vi "Load VI for Subpanel.vi"() -> (2 "VI Path":path, 3 "VI out":refnum<vi>)   [LabVIEW 2021, in "TSC Button Editor.lvclass"]
doc: "This VI loads in the subpanel VI at program start which contains a sample Boolean control.\n\n<b>Code Developed By:</b>\nTechnology Service Corporation\nwww.tsc.com/atcs\n\nDeveloper:\nDaniel Coons"
uses:
  TSC Button Editor.lvclass
  TSC Button Editor.lvclass/TSC Button Editor.ctl
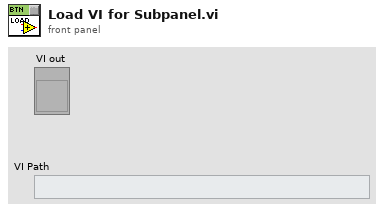
[diagram p1: front panel]
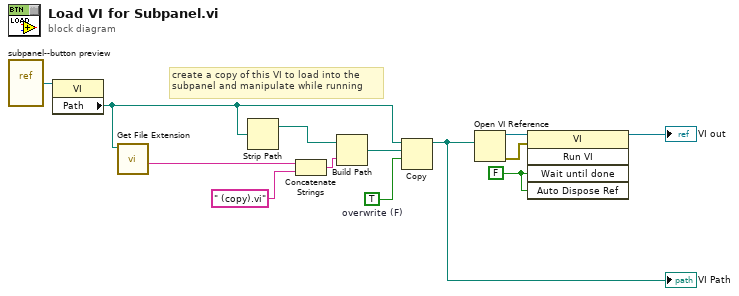
[diagram p0: block diagram]
diagram:
  w4 = TRUE  # overwrite (F)
  w2 = FALSE ("Activate?")
  # "create a copy of this VI to load into the \nsubpanel and manipulate while running"
  n1 = vi-ref "subpanel--button preview.vi"() -> (w3:refnum<vi>)
  n2 = property class="VI"(reference=w3) -> ("Path"=w10:path)  [unwired: 1 in, 2 out]
  n3 = call <vilib>:"Get File Extension.vi"("file"=w10) -> ("filename without extension"=w9:string)  [unwired: 6 in, 4 out]
  n4 = Strip Path(path=w10) -> (stripped path=w7:path)  [unwired: 1 out]
  n5 = Concatenate Strings(w9, " (copy).vi" ("string")) -> (w6:string)
  n6 = Build Path(base path=w7, name or relative path=w6) -> (appended path=w8:path)
  n7 = Copy(9:w4, 10:w8, 11:w10) -> (3:w13:path)  [unwired: 2 in, 2 out]
  "VI Path" <- w13
  n8 = Open VI Reference(vi path=w13) -> (vi reference=w1:refnum<vi>, error out=w12:errorcluster)  [unwired: 5 in]
  n9 = invoke class="VI" method="Run VI"(reference=w1, error in=w12, "Wait until done"=w2, "Auto Dispose Ref"=w2) -> (reference out=→"VI out":refnum<vi>)  [unwired: 1 in, 4 out]
